vi "dynamic.vi"(7 "Boolean":bool, 9 "dynamic":T1, 10 "concatenated":string) -> (1 "dynamic  2":T1, 2 "concatenated string":string)   [LabVIEW 2015]
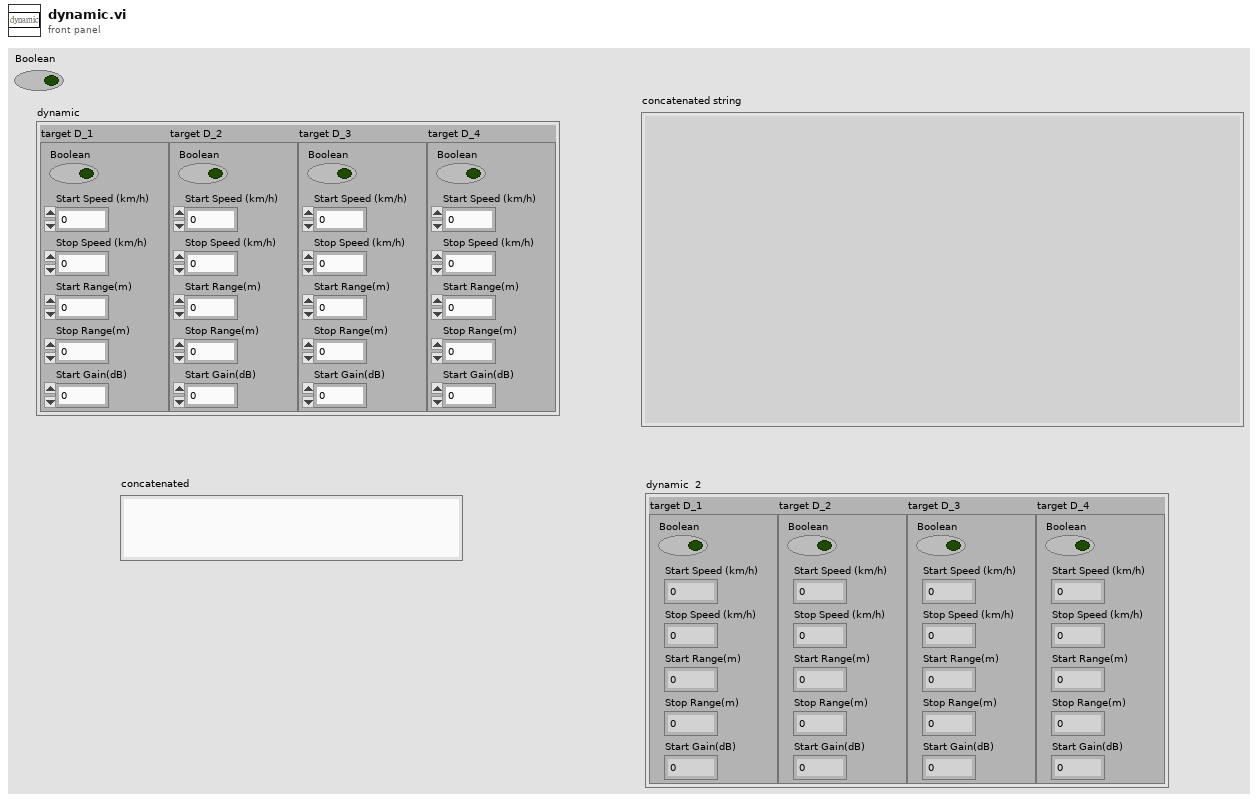
[diagram p1: front panel]
types:
  T1 = cluster{"target D_1":cluster{"Boolean":bool, "Start Speed (km/h)":dbl, "Stop Speed (km/h)":dbl, "Start Range(m)":dbl, "Stop Range(m)":dbl, "Start Gain(dB)":dbl}, "target D_2":cluster{"Boolean":bool, "Start Speed (km/h)":dbl, "Stop Speed (km/h)":dbl, "Start Range(m)":dbl, "Stop Range(m)":dbl, "Start Gain(dB)":dbl}, "target D_3":cluster{"Boolean":bool, "Start Speed (km/h)":dbl, "Stop Speed (km/h)":dbl, "Start Range(m)":dbl, "Stop Range(m)":dbl, "Start Gain(dB)":dbl}, "target D_4":cluster{"Boolean":bool, "Start Speed (km/h)":dbl, "Stop Speed (km/h)":dbl, "Start Range(m)":dbl, "Stop Range(m)":dbl, "Start Gain(dB)":dbl}}
  T2 = cluster{"Boolean":bool, "Start Speed (km/h)":dbl, "Stop Speed (km/h)":dbl, "Start Range(m)":dbl, "Stop Range(m)":dbl, "Start Gain(dB)":dbl}[]
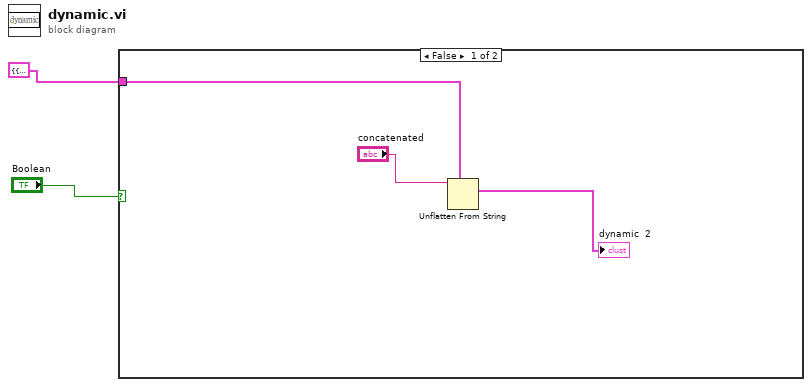
[diagram p0: block diagram]
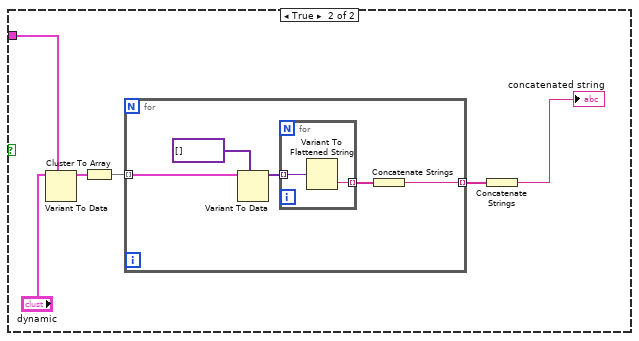
[diagram p2: hidden frame]
diagram:
  n1 = case shown="False" "Boolean" {
    tunnel: T1 {"target D_1"={"Boolean"=FALSE, "Start Speed (km/h)"=0.0, "Stop Speed (km/h)"=0.0, "Start Range(m)"=0.0, "Stop Range(m)"=0.0, "Start Gain(dB)"=0.0}, "target D_2"={"Boolean"=FALSE, "Start Speed (km/h)"=0.0, "Stop Speed (km/h)"=0.0, "Start Range(m)"=0.0, "Stop Range(m)"=0.0, "Start Gain(dB)"=0.0}, "target D_3"={"Boolean"=FALSE, "Start Speed (km/h)"=0.0, "Stop Speed (km/h)"=0.0, "Start Range(m)"=0.0, "Stop Range(m)"=0.0, "Start Gain(dB)"=0.0}, "target D_4"={"Boolean"=FALSE, "Start Speed (km/h)"=0.0, "Stop Speed (km/h)"=0.0, "Start Range(m)"=0.0, "Stop Range(m)"=0.0, "Start Gain(dB)"=0.0}} ("dynamic  2") -> [w4 w7]
    frame False {
      n2 = Unflatten From String(type=w4, binary string="concatenated") -> (value=→"dynamic  2":T1)  [unwired: 3 in, 2 out]
    }
    frame True {
      n3 = Variant To Data(type=w7, Variant="dynamic") -> (data=w11:T1)  [unwired: 1 in, 1 out]
      n4 = Cluster To Array(cluster=w11) -> (array=w10:T2)
      n5 = for {
        tunnel: w10 -> [w14] mode=indexing
        tunnel: [w12] -> w9 mode=indexing
        n6 = Variant To Data(type=variant[] [], Variant=w14) -> (data=w15:variant[])  [unwired: 1 in, 1 out]
        n7 = for {
          tunnel: w15 -> [w18] mode=indexing
          tunnel: [w17] -> w13 mode=indexing
          n8 = Variant To Flattened String(Variant=w18) -> (data string=w17:string)  [unwired: 1 out]
        }
        n9 = Concatenate Strings(w13) -> (w12:string)
      }
      n10 = Concatenate Strings(w9) -> (→"concatenated string":string)
    }
  }
